vi "IsOPCServerRunning.vi"(8 "error in (no error)":errorcluster) -> (0 "error out":errorcluster caption="sortie d'erreur", 1 "NI OPC ON?":bool, 2 "Serveur OPC ModBus ON?":bool)   [LabVIEW 2012]
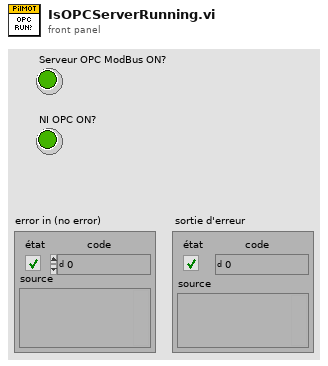
[diagram p1: front panel]
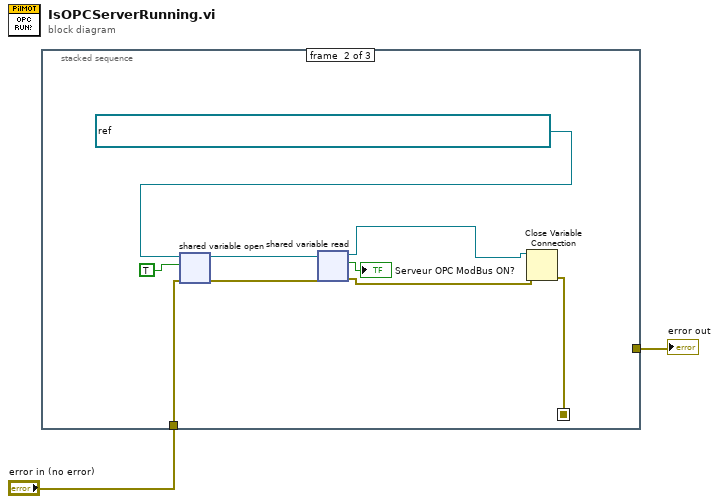
[diagram p0: block diagram]
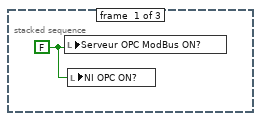
[diagram p2: hidden frame]
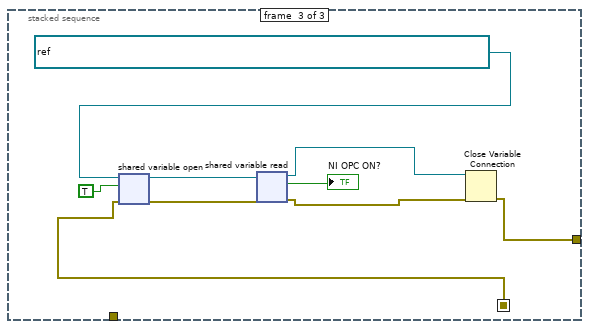
[diagram p3: hidden frame]
diagram:
  n1 = stacked-sequence {
    seq-local: [_ w5 _] -> [_ _ w15]
    tunnel: "error in (no error)" -> [_ w4 _]
    tunnel: [_ _ w14] -> w1
    frame #0 {
      w3 = FALSE
      n2 = local write "Serveur OPC ModBus ON?"(w3) -> ()
      n3 = local write "NI OPC ON?"(w3) -> ()
    }
    frame #1 {
      n4 = shared-variable-open(refnum<k21> "ni.var.psp://localhost/OPC/OPC/NI OPC Client Status/Connected%3F" ("refnum de variable partagée en entrée"), w4, TRUE) -> (w8:refnum<k21>, w9:errorcluster)  [unwired: 1 in]
      n5 = shared-variable-read(w8, w9) -> (w7:refnum<k21>, w6:errorcluster, →"Serveur OPC ModBus ON?":bool)  [unwired: 1 out]
      n6 = Close Variable Connection(8:w6, 11:w7) -> (0:w5:errorcluster)
    }
    frame #2 {
      n7 = shared-variable-open(refnum<k21> "ni.var.psp://localhost/OPC/OPC/NI OPC Client Status/Active%3F" ("refnum de variable partagée en entrée"), w15, TRUE) -> (w18:refnum<k21>, w19:errorcluster)  [unwired: 1 in]
      n8 = shared-variable-read(w18, w19) -> (w17:refnum<k21>, w16:errorcluster, →"NI OPC ON?":bool)  [unwired: 1 out]
      n9 = Close Variable Connection(8:w16, 11:w17) -> (0:w14:errorcluster)
    }
  }
  "error out" <- w1
